vi "Date intrare pentru predictia diabetului.vi"() -> ()   [LabVIEW 2024]
panel:
  out "appended array":dbl[][](array[numeric])
  in  "IMC minim":dbl
  in  "IMC maxim":dbl
  in  "varsta minima":dbl
  in  "varsta maxima":dbl
  in  "insulina minima":dbl
  in  "insulina maxima":dbl
  in  "tensiunea arteriala minima":dbl
  in  "tensiunea arteriala maxima":dbl
  in  "glucoza minima [mg]":dbl
  in  "glucoza maxima [mg]":dbl
  in  "Valori esantion":i32
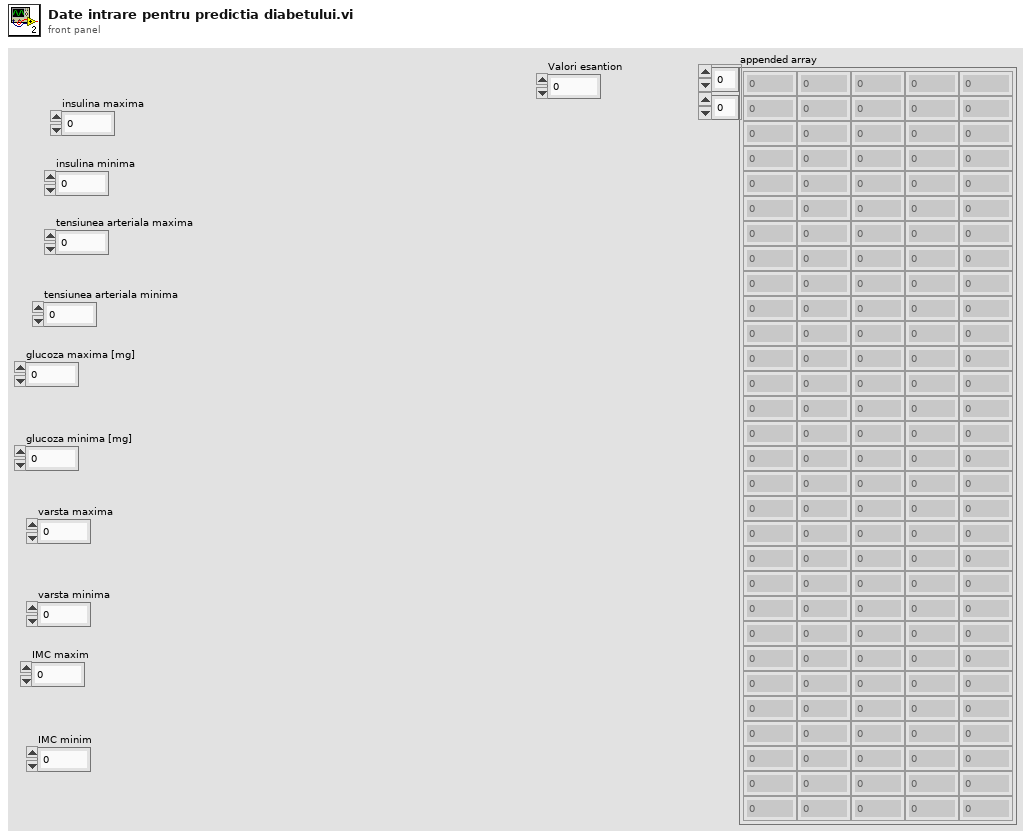
[diagram p1: front panel]
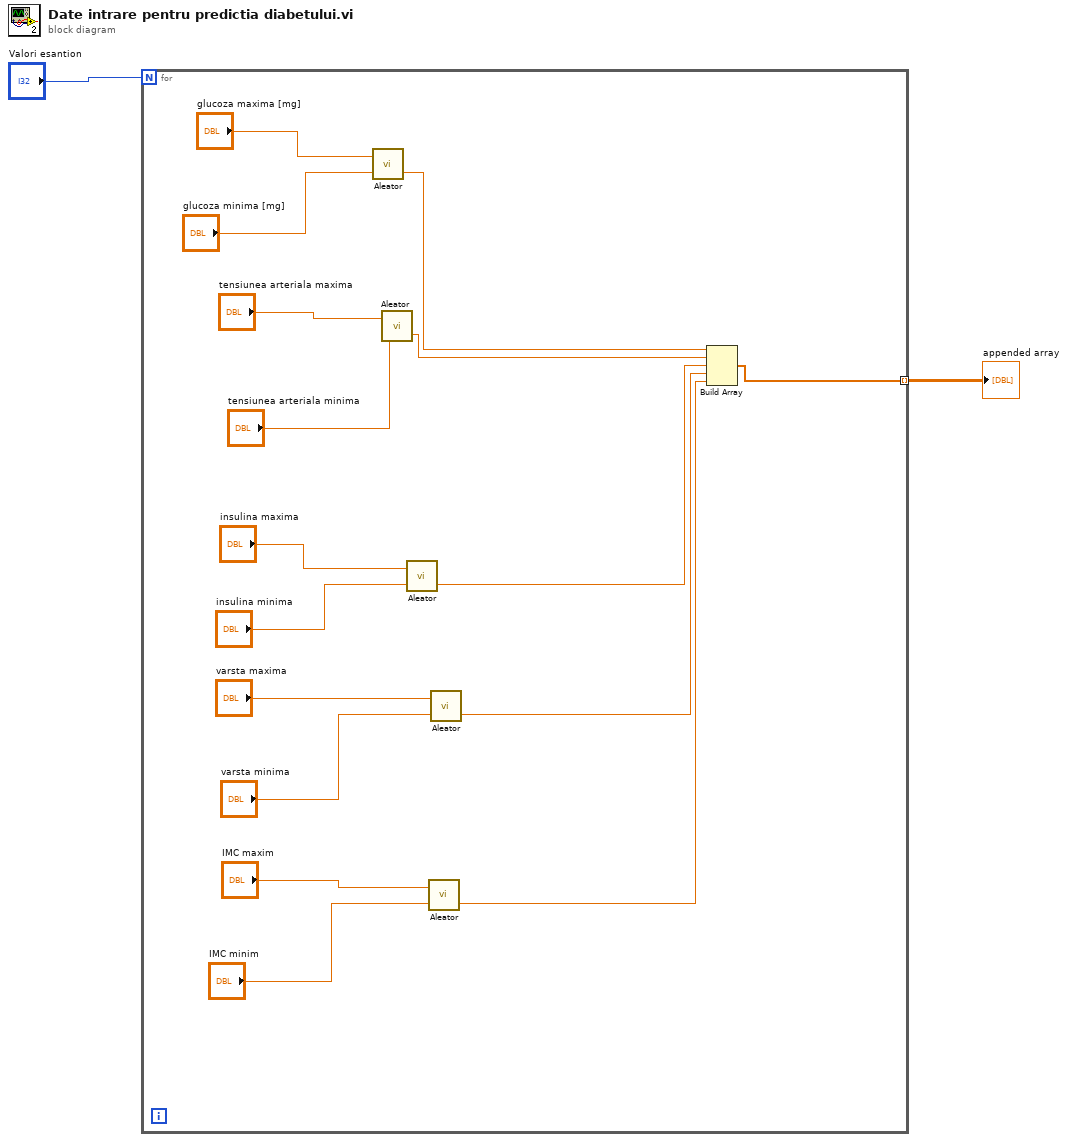
[diagram p0: block diagram]
diagram:
  n1 = for {
    N: "Valori esantion" -> [_]
    tunnel: [w3] -> w1 mode=indexing
    n2 = call "Aleator.vi"("minim"="glucoza minima [mg]", "maxim"="glucoza maxima [mg]") -> ("x val aleatoare"=w8:dbl)  [unwired: 1 in]
    n3 = call "Aleator.vi"("minim"="tensiunea arteriala minima", "maxim"="tensiunea arteriala maxima") -> ("x val aleatoare"=w7:dbl)  [unwired: 1 in]
    n4 = call "Aleator.vi"("minim"="insulina minima", "maxim"="insulina maxima") -> ("x val aleatoare"=w6:dbl)  [unwired: 1 in]
    n5 = call "Aleator.vi"("minim"="IMC minim", "maxim"="IMC maxim") -> ("x val aleatoare"=w4:dbl)  [unwired: 1 in]
    n6 = call "Aleator.vi"("minim"="varsta minima", "maxim"="varsta maxima") -> ("x val aleatoare"=w5:dbl)  [unwired: 1 in]
    n7 = Build Array(w8, w7, w6, w5, w4) -> (w3:dbl[])
  }
  "appended array" <- w1
